vi "Get IP Reg Types.vi"(10 "Version":T1, 11 "Digital Pattern Generation in":refnum<class "Digital Pattern Generation.lvclass">) -> (2 "IP Regs":variant[](array[variant]), 3 "Digital Pattern Generation out":refnum<class "Digital Pattern Generation.lvclass">)   [LabVIEW 2013, in "Digital Pattern Generation.lvclass"]
uses:
  Digital Pattern Generation.lvclass
  Bitfile Major Version.ctl
  Engine Simulation Session.lvclass
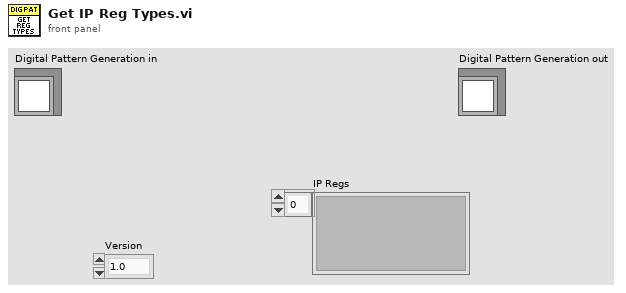
[diagram p1: front panel]
types:
  T1 = typedef "Engine Simulation Session.lvclass/Bitfile Major Version.ctl" = enum16{"1.0", "1.1", "1.2", "1.3"}
  T2 = cluster{"address":fxp<+,11,11>, "done":bool, "angle":u16}
  T3 = cluster{"edge 1":u16, "edge 2":u16, "cycle angle":bool, "enabled":bool, "first falling":bool}
  T4 = cluster{"edge 1":u16, "edge 2":u16, "cycle angle":bool, "enabled":bool, "first falling":bool, "fault":bool, "fault wrap":bool, "fault value":bool, "fault count":fxp<+,4,4>, "use fault count":bool}
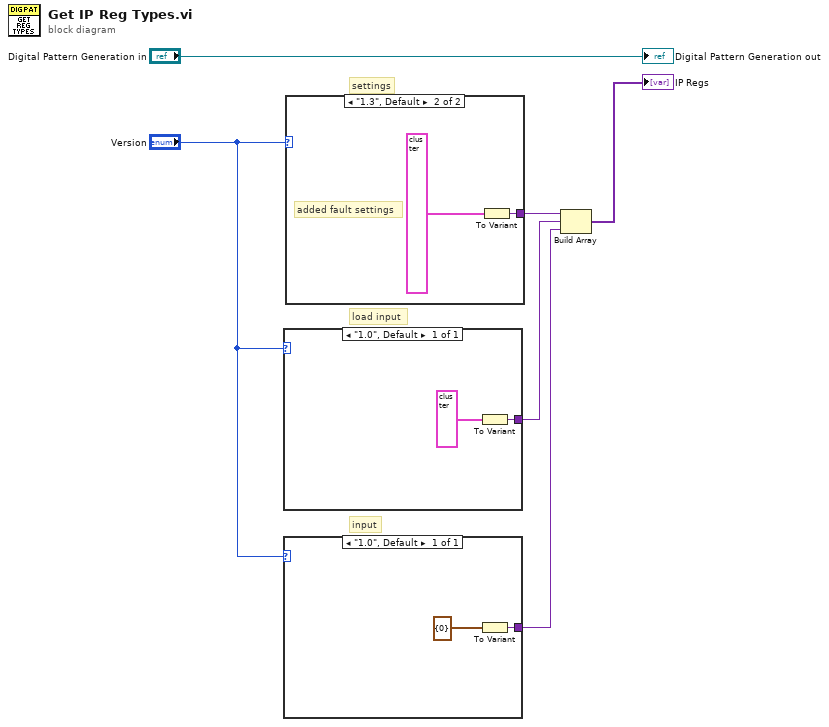
[diagram p0: block diagram]
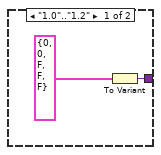
[diagram p2: hidden frame]
diagram:
  # "input"
  # "load input"
  # "settings"
  n1 = case shown="\"1.0\", Default" "Version" {
    tunnel: [w8] -> w3
    frame "1.0", Default {
      n2 = To Variant(anything=T2 {"address"=0.0, "done"=FALSE, "angle"=0}) -> (Variant=w8:variant)
    }
  }
  n3 = case shown="\"1.0\", Default" "Version" {
    tunnel: [w10] -> w2
    frame "1.0", Default {
      n4 = To Variant(anything=cluster{"Offset":i16} {"Offset"=0}) -> (Variant=w10:variant)
    }
  }
  n5 = case shown="\"1.3\", Default" "Version" {
    tunnel: [w12 w14] -> w4
    frame "1.0".."1.2" {
      n6 = To Variant(anything=T3 {"edge 1"=0, "edge 2"=0, "cycle angle"=FALSE, "enabled"=FALSE, "first falling"=FALSE} ("settings")) -> (Variant=w12:variant)
    }
    frame "1.3", Default {
      # "added fault settings"
      n7 = To Variant(anything=T4 {"edge 1"=0, "edge 2"=0, "cycle angle"=FALSE, "enabled"=FALSE, "first falling"=FALSE, "fault"=FALSE, "fault wrap"=FALSE, "fault value"=FALSE, "fault count"=0.0, "use fault count"=FALSE} ("settings")) -> (Variant=w14:variant)
    }
  }
  n8 = Build Array(w4, w3, w2) -> (→"IP Regs":variant[])
  "Digital Pattern Generation out" <- "Digital Pattern Generation in"
